vi "ModbusTest.vi"() -> ()   [LabVIEW 2011]
uses:
  <vilib>/NI/Modbus Library/API/Wrapper/API Main.lvlib
  <vilib>/NI/Modbus Library/API/Wrapper/Create Serial Master.vi
  <vilib>/NI/Modbus Library/API/Master/Modbus Master.lvclass
panel:
  out "ReadHRegsError":errorcluster
  out "HoldingRegsRead":u16[](array[numeric])
  in  "Cantidad":u16 min=1
  in  "DireccionInicial":u16
  out "ErrorCloseVISA":errorcluster
  in  "stop":bool
  in  "Habilitar lectura":bool
  in  "read-write operation timeout":i32=1500
  out "serial master instance":refnum<class "Modbus Master.lvclass">
  in  "parity (even)":u16(ring) items=["None", "Odd", "Even", "Mark", "Space"]
  in  "unit ID":u8=2
  in  "serial type":enum16{"RTU", "ASCII"}(ring)
  in  "VISA resource name":refnum<visa-resource-name>
  in  "baud rate":u32=9600
  out "Error MB Instance":errorcluster
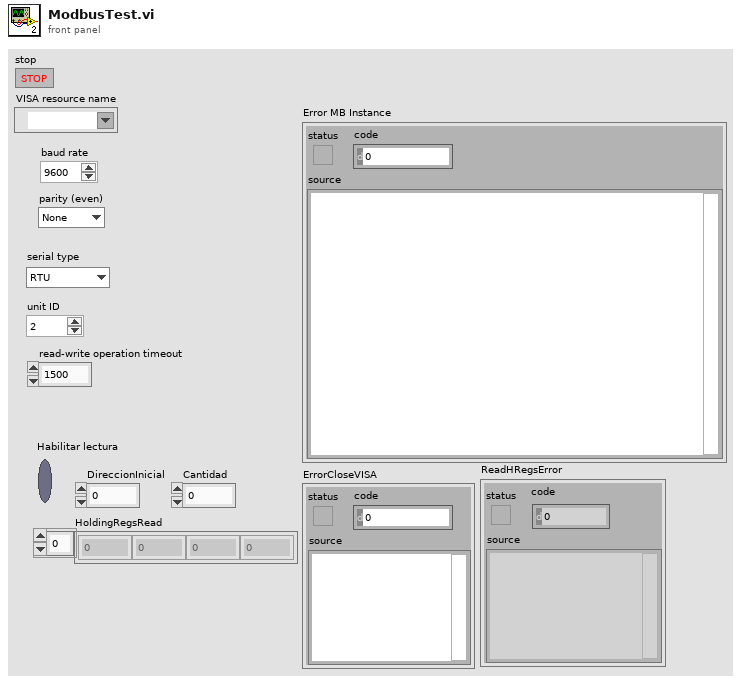
[diagram p1: front panel]
types:
  T1 = enum8{"Enabled", "Disabled", "Disabled and Grayed Out"}
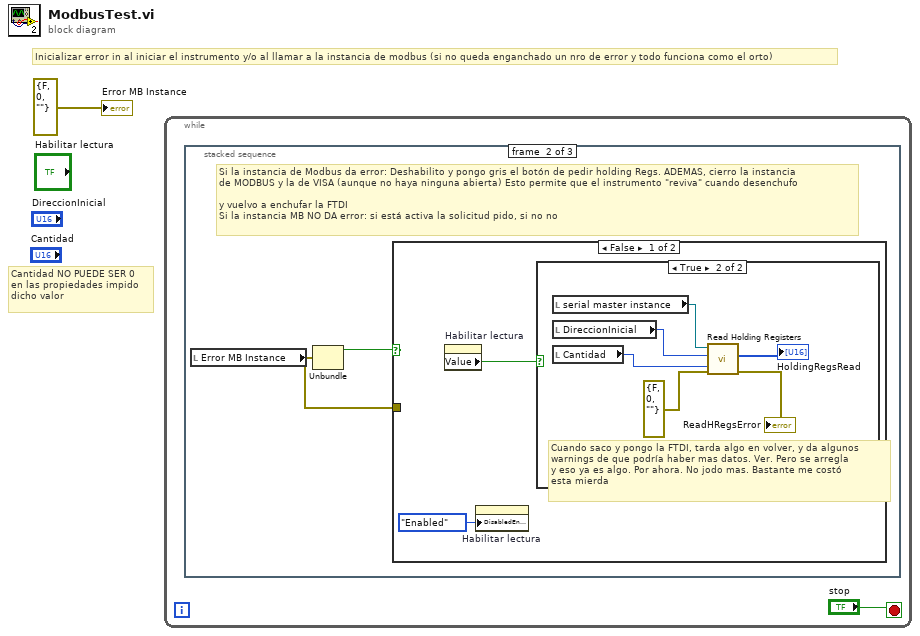
[diagram p0: block diagram]
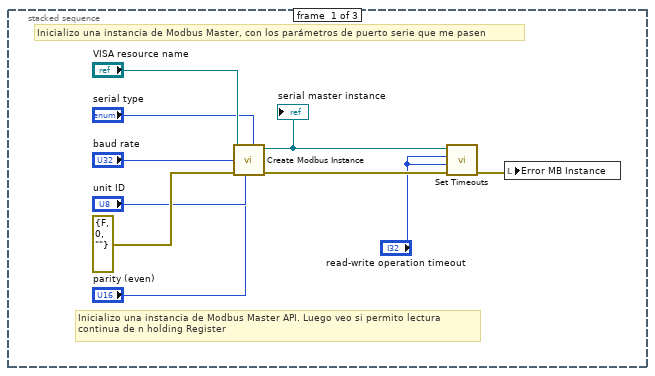
[diagram p2: hidden frame]
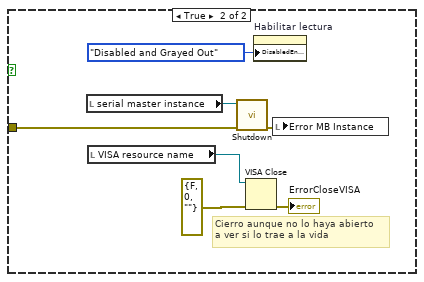
[diagram p4: hidden frame]
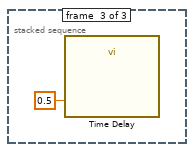
[diagram p5: hidden frame]
diagram:
  # "Cantidad NO PUEDE SER 0 \nen las propiedades impido\ndicho valor"
  # "Inicializar error in al iniciar el instrumento y/o al llamar a la instancia de modbus (si no queda enganchado un nro de error y todo funciona como el orto)"
  n1 = while {
    stop <- "stop" stop-if-true
    n2 = stacked-sequence {
      frame #0 {
        # "Inicializo una instancia de Modbus Master, con los parámetros de puerto serie que me pasen"
        # "Inicializo una instancia de Modbus Master API. Luego veo si permito lectura \ncontinua de n holding Register"
        n3 = call-poly <vilib>:"Create Modbus Instance.vi"("serial type"="serial type", "parity (even)"="parity (even)", "unit ID"="unit ID", "error in"=errorcluster {"status"=FALSE, "code"=0, "source"=""}, "baud rate"="baud rate", "VISA resource name"="VISA resource name") -> ("error out"=w5:errorcluster, "serial master instance"=w6:refnum<class "Modbus Master.lvclass">)  [unwired: 4 in]
        "serial master instance" <- w6
        n4 = call <vilib>:"Set Timeouts.vi"("error in"=w5, "write operation timeout"="read-write operation timeout", "read operation timeout"="read-write operation timeout", "Modbus master in"=w6) -> ("error out"=w4:errorcluster)  [unwired: 6 in, 1 out]
        n5 = local write "Error MB Instance"(w4) -> ()
      }
      frame #1 {
        # "Si la instancia de Modbus da error: Deshabilito y pongo gris el botón de pedir holding Regs. ADEMAS, cierro la instancia \nde MODBUS y la de VISA (aunque no haya ninguna abierta) Esto permite que el instrumento \"reviva\" cuando desenchufo \n\ny vuelvo a enchufar la FTDI\nSi la instancia MB NO DA error: si está activa la solicitud pido, si no no"
        n6 = local read "Error MB Instance"() -> (w13:errorcluster)
        n7 = Unbundle(w13) -> ("status"=w14:bool)  [unwired: 2 out]
        n8 = case shown="False" w14 {
          tunnel: w13 -> [_ w27]
          frame False {
            n9 = property on="Habilitar lectura" class="Bool (strict)"() -> ("Value"=w16:bool)  [unwired: 2 in, 2 out]
            n10 = property on="Habilitar lectura" class="Bool (strict)"("DisabledEnum"=T1."Enabled" ("Disabled")) -> ()  [unwired: 2 in, 2 out]
            n11 = case shown="True" w16 {
              frame False {
              }
              frame True {
                # "Cuando saco y pongo la FTDI, tarda algo en volver, y da algunos\nwarnings de que podría haber mas datos. Ver. Pero se arregla\ny eso ya es algo. Por ahora. No jodo mas. Bastante me costó\nesta mierda"
                n12 = local read "serial master instance"() -> (w19:refnum<class "Modbus Master.lvclass">)
                n13 = local read "DireccionInicial"() -> (w20:u16)
                n14 = local read "Cantidad"() -> (w21:u16)
                n15 = call-dynamic "Read Holding Registers.vi"("error in"=errorcluster {"status"=FALSE, "code"=0, "source"=""}, "number of inputs"=w21, "starting address"=w20, "Modbus master in"=w19) -> ("error out"=→"ReadHRegsError":errorcluster, "register values"=→"HoldingRegsRead":u16[])  [unwired: 5 in, 1 out]
              }
            }
          }
          frame True {
            # "Cierro aunque no lo haya abierto\na ver si lo trae a la vida"
            n16 = local read "serial master instance"() -> (w28:refnum<class "Modbus Master.lvclass">)
            n17 = local read "VISA resource name"() -> (w25:refnum<visa-resource-name>)
            n18 = call-dynamic "Shutdown.vi"("error in"=w27, "Modbus master in"=w28) -> ("error out"=w26:errorcluster)  [unwired: 9 in]
            n19 = VISA Close(VISA resource name=w25, error in (no error)=errorcluster {"status"=FALSE, "code"=0, "source"=""}) -> (error out=→"ErrorCloseVISA":errorcluster)
            n20 = property on="Habilitar lectura" class="Bool (strict)"("DisabledEnum"=T1."Disabled and Grayed Out" ("Disabled")) -> ()  [unwired: 2 in, 2 out]
            n21 = local write "Error MB Instance"(w26) -> ()
          }
        }
      }
      frame #2 {
        n22 = call "Time Delay"("Delay Time (s)"=0.5) -> ()  [unwired: 10 in, 1 out]
      }
    }
  }
  "Error MB Instance" <- errorcluster {"status"=FALSE, "code"=0, "source"=""} ("error in")
